vi "get_depth_imaq.vi"(8 "error in":errorcluster, 9 "Image Resource In":T2, 10 "fmt":T1(ring), 11 "index":i32) -> (0 "error out":errorcluster, 1 "Image Resource Out":T2)   [LabVIEW 2017, in "libfreenect.lvlib"]
uses:
  libfreenect.lvlib
  <vilib>/vision/Image Controls.llb/IMAQ Image.ctl
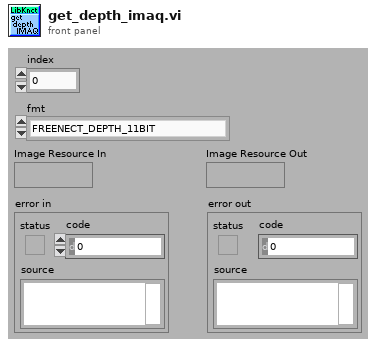
[diagram p1: front panel]
types:
  T1 = enum16{"FREENECT_DEPTH_11BIT", "FREENECT_DEPTH_10BIT", "FREENECT_DEPTH_11BIT_PACKED", "FREENECT_DEPTH_10BIT_PACKED"}
  T2 = typedef "IMAQ Image.ctl" = refnum<image>
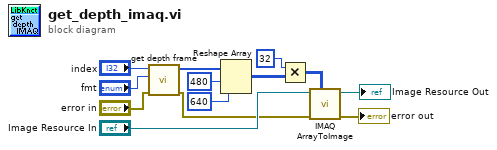
[diagram p0: block diagram]
diagram:
  n1 = call "get depth frame.vi"("error in (no error)"="error in", "fmt"="fmt", "index"="index") -> ("error out"=w4:errorcluster, "Destination"=w11:u16[])  [unwired: 7 out]
  n2 = Reshape Array(w11, 480 ("dimension size"), 640 ("dimension size")) -> (w3:u16[][])
  n3 = Multiply(x=32, y=w3) -> (x*y=w1:i32[][])
  n4 = call "IMAQ ArrayToImage"("Image Pixels (U16)"=w1, "error in (no error)"=w4, "Image"="Image Resource In") -> ("error out"=→"error out":errorcluster, "Image Out"=→"Image Resource Out":T2)  [unwired: 3 in, 4 out]
